vi "construct.vi"(8 "error in (no error)":errorcluster, 9 "configuration name":string, 10 "load config file?":bool=TRUE, 11 "SignalReaderDL091205FPGA in":refnum<class "SignalReaderDL091205FPGA.lvclass">) -> (0 "error out":errorcluster, 3 "SignalReaderDL091205FPGA out":refnum<class "SignalReaderDL091205FPGA.lvclass">)   [LabVIEW 2010, in "SignalReaderDL091205FPGA.lvclass"]
uses:
  SignalReaderDL091205FPGA.lvclass
  GenericSignalReader/GenericSignalReader/GenericSignalReader.lvclass
  SignalReaderDL091205FPGA.lvclass/SignalReaderDL091205FPGA.ctl
  common/classes/GenericComponent/GenericComponent/GenericComponent.lvclass
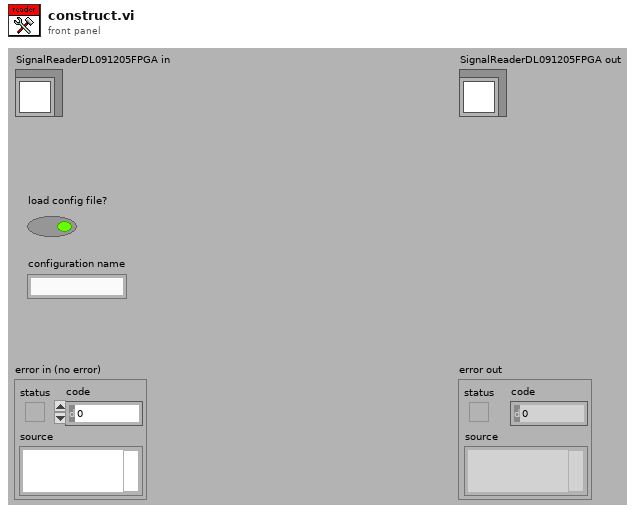
[diagram p1: front panel]
types:
  T1 = typedef "plugin_specification.ctl" = cluster{"class path":string, "configuration":string, "label":string, "settings name":string}
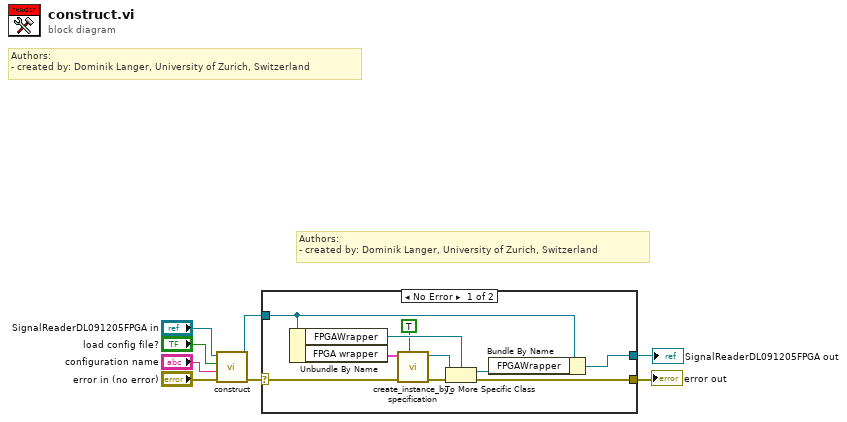
[diagram p0: block diagram]
diagram:
  # "Authors: \n- created by: Dominik Langer, University of Zurich, Switzerland"
  # "Authors: \n- created by: Dominik Langer, University of Zurich, Switzerland"
  n1 = call-parent "construct.vi"("error in (no error)"="error in (no error)", "configuration name"="configuration name", "load config file?"="load config file?", "GenericPlugin in"="SignalReaderDL091205FPGA in") -> ("error out"=w4:errorcluster, "GenericPlugin out"=w3:refnum<class "SignalReaderDL091205FPGA.lvclass">)  [unwired: 6 in]
  n2 = case shown="No Error" w4 {
    selector: w4 -> [w15 w20]
    tunnel: w3 -> [w18 w19]
    tunnel: [w10 w20] -> w2
    tunnel: [w17 w19] -> w1
    frame No Error {
      n3 = Unbundle By Name(w18) -> ("FPGAWrapper"=w14:refnum<class "GenericFPGAWrapper.lvclass">, "FPGA wrapper"=w16:T1)
      n4 = call "create_instance_by_specification.vi"("call constructor?"=TRUE, "error in (no error)"=w15, "component specification"=w16) -> ("error out"=w12:errorcluster, "GenericPlugin out"=w13:refnum<class "GenericComponent.lvclass">)  [unwired: 6 in, 1 out]
      n5 = To More Specific Class(target class=w14, reference=w13, error in=w12) -> (specific class reference=w11:refnum<class "GenericFPGAWrapper.lvclass">, error out=w10:errorcluster)
      n6 = Bundle By Name(cluster=w18, "FPGAWrapper"=w11) -> (w17:refnum<class "SignalReaderDL091205FPGA.lvclass">)
    }
    frame Error {
    }
  }
  "error out" <- w2
  "SignalReaderDL091205FPGA out" <- w1
